vi "scanControlView.vi"(10 "UserEvents in":refnum<class "UserEvents.lvclass">) -> ()   [LabVIEW 2015, in "FAMTViews.lvlib"]
uses:
  FAMTViews.lvlib
  UserEvents/UserEvents.lvclass
  Typedefs/Test Values.ctl
  <userlib>/Common/ILC/Configuration/Scan Rates.ctl
  Typedefs/Waveform.ctl
  CommandFactory/CommandFactory.lvclass
  UserEvents/UserEvents.lvclass/UserEvents.ctl
  Typedefs/StateSelector.ctl
  Commands/StartOpenLoopScan/StartOpenLoopScan.lvclass
  Typedefs/Scan Settings.ctl
  Commands/StartOpenLoopScan/StartOpenLoopScan.lvclass/StartOpenLoopScan.ctl
  Typedefs/CommandSelector.ctl
  Typedefs/FAMTTypedefs.lvlib
  <userlib>/Common/ILC/Configuration/ILCConfiguration.lvlib
panel:
  in  "Settling Time":dbl[unit]=1.0
  in  "Hold Time":dbl[unit]
  in  "Ramp Time":dbl[unit]
  in  "Notes":string
  in  "Scan Name":string
  in  "Operator":string
  in  "Waveform":T1
  in  "F1":dbl[unit]=1.0
  in  "F2":dbl[unit]=10.0
  in  "Duty Cycle":dbl=0.5
  in  "Frequency":dbl[unit]=2.0
  in  "Offset":dbl[unit]
  in  "Amplitude":dbl[unit]=1.0
  in  "Iterations":dbl=5.0
  in  "Samples":u32=1000
  in  "Rate Scan Settings":T2[](array[typedef])=[enum."480"]
  in  "Amplitude Scan Settings":T3={"Start Value"=1.0, "Stop Value"=1.0, "Steps"=1} {"Stop Value" format="%.3f"; "Start Value" format="%.3f"}
  in  "cancelOpenLoopScanIsTrue":bool
  in  "startOpenLoopScanIsTrue":bool
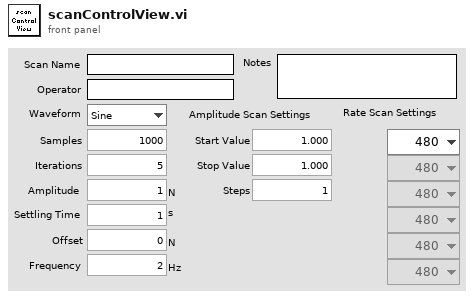
[diagram p1: front panel]
types:
  T1 = typedef "FAMTTypedefs.lvlib/Waveform.ctl" = enum16{"Sine", "Triangle", "Square", "Sawtooth", "Chirp", "Gaussian", "Trapezoid"}
  T2 = typedef "ILCCommon.lvlib/ILCConfiguration.lvlib/Scan Rates.ctl" = enum16{"50", "60", "100", "120", "200", "240", "300", "400", "480", "600", "1200", "2400", "4800"}
  T3 = typedef "FAMTTypedefs.lvlib/Test Values.ctl" = cluster{"Start Value":dbl, "Stop Value":dbl, "Steps":u16}
  T4 = typedef "FAMTTypedefs.lvlib/PubDataEvents.ctl" = cluster{"State":refnum<user-event>, "ErrorCode":refnum<user-event>, "ADC Outputs":refnum<user-event>, "InputData":refnum<user-event>, "ControllerData":refnum<user-event>, "TestStatus":refnum<user-event>, "LogPath":refnum<user-event>, "ILC Outputs":refnum<user-event>, "Scan Progress":refnum<user-event>}
  T5 = typedef "FAMTTypedefs.lvlib/SubDataEvents.ctl" = cluster{"Command":refnum<user-event>}
  T6 = cluster{"Event Registration Refnum":refnum<event-registration>}
  T7 = typedef "FAMTTypedefs.lvlib/StateSelector.ctl" = enum16{"OfflineState", "FaultState", "StandbyState", "DisabledState", "EnabledState", "WaitForUserInputState", "PerformOpenLoopScanState", "PerformPreScanHoldState", "PerformPostScanHoldState", "PerformScanState"}
  T8 = typedef "FAMTTypedefs.lvlib/Scan Settings.ctl" = cluster{"Amplitude Scan Settings":T3, "Rate Scan Settings":T2[], "Sample Count":u32, "Iterations":dbl, "Amplitude":dbl[unit], "Offset":dbl[unit], "Frequency":dbl[unit], "Waveform":T1, "F1":dbl[unit], "F2":dbl[unit], "Duty Cycle":dbl, "ILC Rate":dbl[unit], "Operator":string, "Scan Name":string, "Notes":string, "Ramp Time":dbl[unit], "Hold Time":dbl[unit], "Settling Time":dbl[unit]}
  T9 = typedef "FAMTTypedefs.lvlib/CommandSelector.ctl" = enum16{"Start", "Enable", "Disable", "Standby", "Shutdown", "Update"}
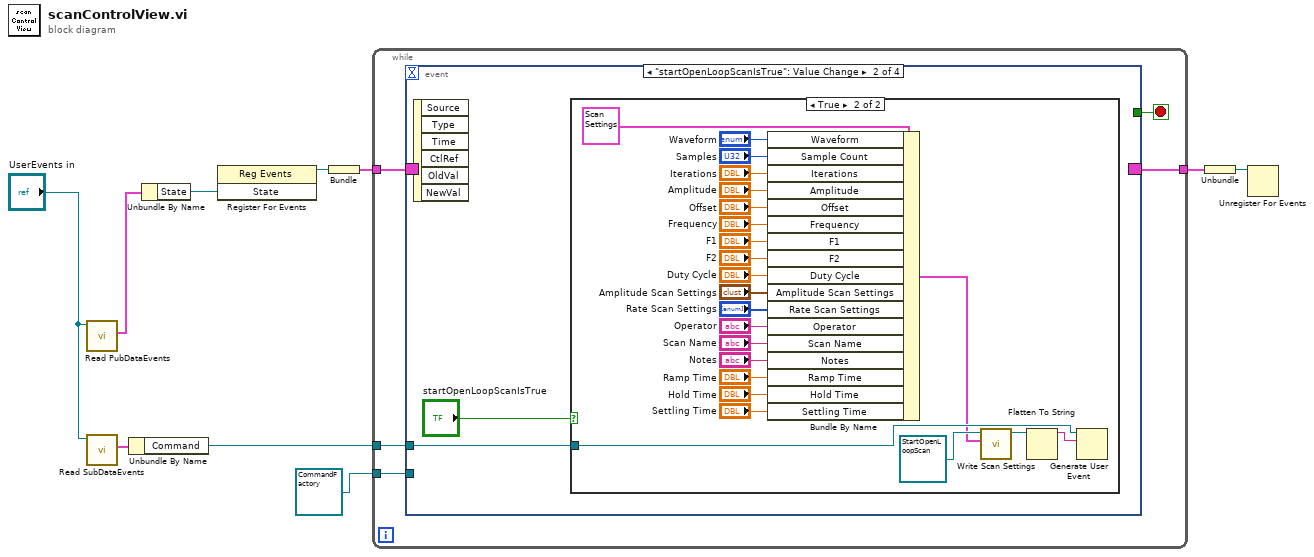
[diagram p0: block diagram]
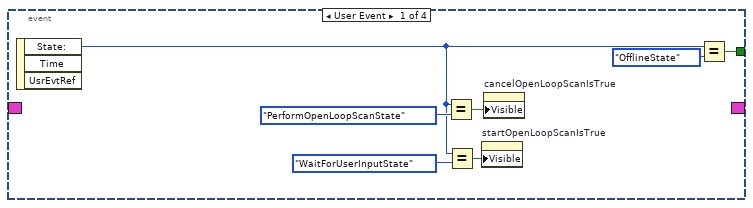
[diagram p2: hidden frame]
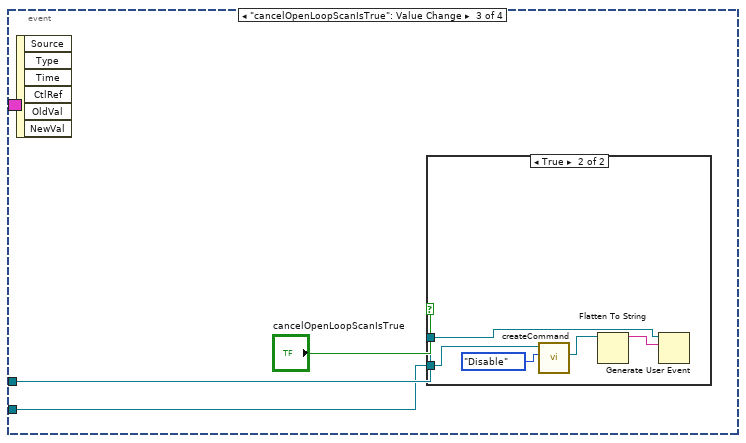
[diagram p4: hidden frame]
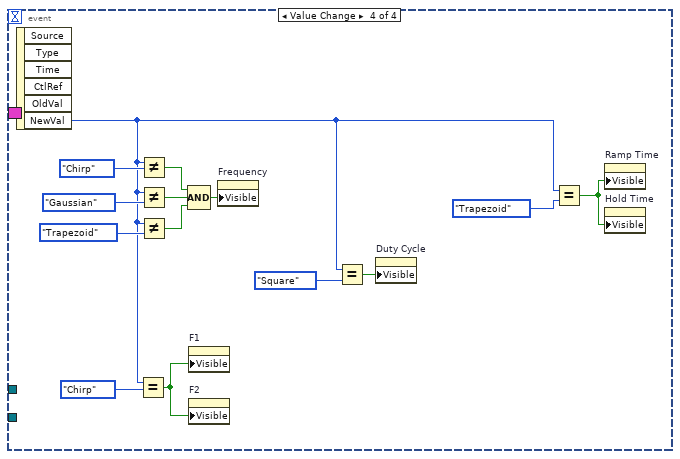
[diagram p6: hidden frame]
diagram:
  n1 = call "Read PubDataEvents.vi"("UserEvents in"="UserEvents in") -> ("PubDataEvents"=w10:T4)  [unwired: 9 in, 1 out]
  n2 = call "Read SubDataEvents.vi"("UserEvents in"="UserEvents in") -> ("SubDataEvents"=w4:T5)  [unwired: 9 in, 1 out]
  n3 = Unbundle By Name(w4) -> ("Command"=w2:refnum<user-event>)
  n4 = Unbundle By Name(w10) -> ("State"=w9:refnum<user-event>)
  n5 = register-events(w9) -> (reference out=w8:refnum<event-registration>)  [unwired: 2 in, 1 out]
  n6 = Bundle("Event Registration Refnum"=w8) -> (w5:T6)  [unwired: 1 in]
  n7 = while {
    tunnel: w5 -> [w15]
    tunnel: [w14] -> w6
    tunnel: w2 -> [w12]
    tunnel: refnum<class "CommandFactory.lvclass"> refnum ("CommandFactory.lvclass") -> [w11]
    stop <- w13 stop-if-true
    n8 = event shown="[1] \"startOpenLoopScanIsTrue\": Value Change" {
      selector: w15 -> [_ _ _ _]
      dyn-events: [_ _ _ _] -> w14
      timeout: _ -> [_ _ _ _]
      tunnel: [w21 _ _ _] -> w13
      tunnel: w12 -> [_ w23 w49 _]
      tunnel: w11 -> [_ _ w48 _]
      event User Event {
        n9 = event-data() -> ("State:"=w18:T7)  [unwired: 1 in, 2 out]
        n10 = Equal?(x=w18, y=StateSelector."PerformOpenLoopScanState") -> (x = y?=w17:bool)
        n11 = Equal?(x=w18, y=StateSelector."WaitForUserInputState") -> (x = y?=w16:bool)
        n12 = property on="startOpenLoopScanIsTrue" class="Bool"("Visible"=w16) -> ()  [unwired: 2 in, 2 out]
        n13 = property on="cancelOpenLoopScanIsTrue" class="Bool"("Visible"=w17) -> ()  [unwired: 2 in, 2 out]
        n14 = Equal?(x=w18, y=StateSelector."OfflineState") -> (x = y?=w21:bool)
      }
      event "startOpenLoopScanIsTrue": Value Change {
        n15 = event-data() -> ()  [unwired: 1 in, 6 out]
        n16 = case shown="True" "startOpenLoopScanIsTrue" {
          tunnel: w23 -> [_ w46]
          frame False {
          }
          frame True {
            n17 = Bundle By Name(cluster=T8 {"Amplitude Scan Settings"={"Start Value"=1.0, "Stop Value"=1.0, "Steps"=2}, "Rate Scan Settings"=[], "Sample Count"=0, "Iterations"=0.0, "Amplitude"=0.0, "Offset"=0.0, "Frequency"=0.0, "Waveform"=enum."Sine", "F1"=0.0, "F2"=0.0, "Duty Cycle"=0.0, "ILC Rate"=0.0, "Operator"="", "Scan Name"="", "Notes"="", "Ramp Time"=0.0, "Hold Time"=0.0, "Settling Time"=0.0} ("Scan Settings"), "Waveform"="Waveform", "Sample Count"="Samples", "Iterations"="Iterations", "Amplitude"="Amplitude", "Offset"="Offset", "Frequency"="Frequency", "F1"="F1", "F2"="F2", "Duty Cycle"="Duty Cycle", "Amplitude Scan Settings"="Amplitude Scan Settings", "Rate Scan Settings"="Rate Scan Settings", "Operator"="Operator", "Scan Name"="Scan Name", "Notes"="Notes", "Ramp Time"="Ramp Time", "Hold Time"="Hold Time", "Settling Time"="Settling Time") -> (w31:T8)
            n18 = call "Write Scan Settings.vi"("Scan Settings"=w31, "StartOpenLoopScan in"=refnum<class "StartOpenLoopScan.lvclass"> refnum ("StartOpenLoopScan.lvclass")) -> ("StartOpenLoopScan out"=w44:refnum<class "StartOpenLoopScan.lvclass">)  [unwired: 9 in]
            n19 = Flatten To String(anything=w44) -> (data string=w47:string)  [unwired: 3 in, 2 out]
            n20 = Generate User Event(user event=w46, event data cluster=w47) -> ()  [unwired: 2 in, 2 out]
          }
        }
      }
      event "cancelOpenLoopScanIsTrue": Value Change {
        n21 = event-data() -> ()  [unwired: 1 in, 6 out]
        n22 = case shown="True" "cancelOpenLoopScanIsTrue" {
          tunnel: w49 -> [_ w54]
          tunnel: w48 -> [_ w51]
          frame False {
          }
          frame True {
            n23 = call-dynamic "createCommand.vi"("Command"=CommandSelector."Disable", "CommandFactory in"=w51) -> ("command"=w52:refnum<class "Command.lvclass">)  [unwired: 7 in, 2 out]
            n24 = Flatten To String(anything=w52) -> (data string=w55:string)  [unwired: 3 in, 2 out]
            n25 = Generate User Event(user event=w54, event data cluster=w55) -> ()  [unwired: 2 in, 2 out]
          }
        }
      }
      event Value Change {
        n26 = event-data() -> ("NewVal"=w57:T1)  [unwired: 1 in, 5 out]
        n27 = Equal?(x=w57, y=Waveform."Chirp") -> (x = y?=w67:bool)
        n28 = Not Equal?(x=w57, y=Waveform."Chirp") -> (x != y?=w62:bool)
        n29 = Not Equal?(x=w57, y=Waveform."Gaussian") -> (x != y?=w61:bool)
        n30 = Not Equal?(x=w57, y=Waveform."Trapezoid") -> (x != y?=w60:bool)
        n31 = Compound Arithmetic op=AND(w62, w61, w60) -> (w59:bool)
        n32 = property on="F1" class="DigNum (strict)"("Visible"=w67) -> ()  [unwired: 2 in, 2 out]
        n33 = property on="F2" class="DigNum (strict)"("Visible"=w67) -> ()  [unwired: 2 in, 2 out]
        n34 = property on="Frequency" class="DigNum (strict)"("Visible"=w59) -> ()  [unwired: 2 in, 2 out]
        n35 = Equal?(x=w57, y=Waveform."Square") -> (x = y?=w65:bool)
        n36 = property on="Duty Cycle" class="DigNum (strict)"("Visible"=w65) -> ()  [unwired: 2 in, 2 out]
        n37 = Equal?(x=w57, y=Waveform."Trapezoid") -> (x = y?=w56:bool)
        n38 = property on="Ramp Time" class="DigNum (strict)"("Visible"=w56) -> ()  [unwired: 2 in, 2 out]
        n39 = property on="Hold Time" class="DigNum (strict)"("Visible"=w56) -> ()  [unwired: 2 in, 2 out]
      }
    }
  }
  n40 = Unbundle(w6) -> ("Event Registration Refnum"=w7:refnum<event-registration>)
  n41 = Unregister For Events(event registration refnum=w7) -> ()  [unwired: 1 in, 1 out]
